vi "get_total_number_of_pixels_per_line.vi"(8 "error in (no error)":errorcluster, 11 "DL090201FrameScanTrajectory in":refnum<class "TrajectoryDL090201FrameScan.lvclass">) -> (0 "error out":errorcluster, 2 "total number of pixels per line":i32, 3 "DL090201FrameScanTrajectory out":refnum<class "TrajectoryDL090201FrameScan.lvclass">)   [LabVIEW 2010, in "TrajectoryDL090201FrameScan.lvclass"]
uses:
  TrajectoryDL090201FrameScan.lvclass
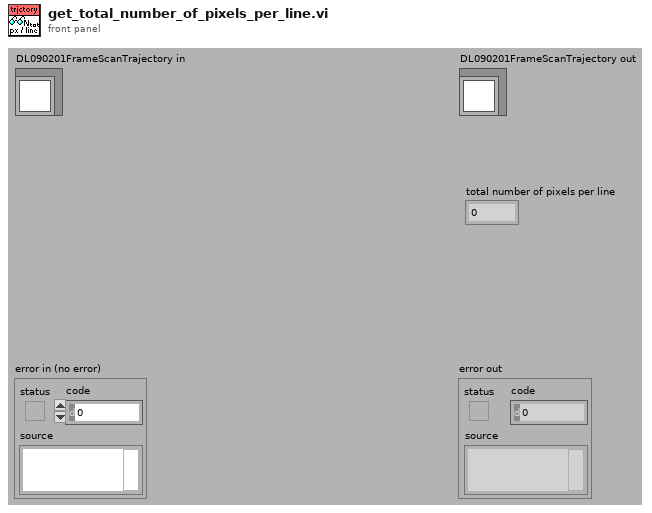
[diagram p1: front panel]
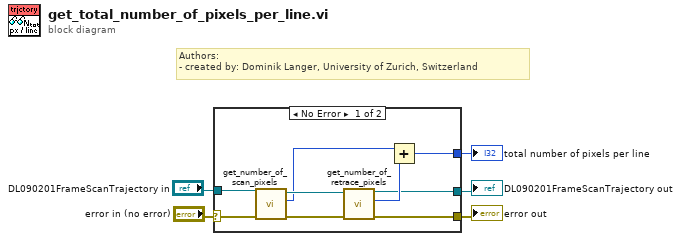
[diagram p0: block diagram]
diagram:
  # "Authors: \n- created by: Dominik Langer, University of Zurich, Switzerland"
  n1 = case shown="No Error" "error in (no error)" {
    selector: "error in (no error)" -> [w13 w16]
    tunnel: [w12 w16] -> w4
    tunnel: [w6 w15] -> w2
    tunnel: "DL090201FrameScanTrajectory in" -> [w7 w15]
    tunnel: [w8 _] -> w1
    frame No Error {
      n2 = call "get_number_of_scan_pixels.vi"("error in (no error)"=w13, "DL090201FrameScanTrajectory in"=w7) -> ("error out"=w14:errorcluster, "number of scan pixels"=w10:i32, "DL090201FrameScanTrajectory out"=w11:refnum<class "TrajectoryDL090201FrameScan.lvclass">)  [unwired: 7 out]
      n3 = call "get_number_of_retrace_pixels.vi"("error in (no error)"=w14, "DL090201FrameScanTrajectory in"=w11) -> ("error out"=w12:errorcluster, "number of retrace pixels"=w9:i32, "DL090201FrameScanTrajectory out"=w6:refnum<class "TrajectoryDL090201FrameScan.lvclass">)  [unwired: 7 out]
      n4 = Add(x=w10, y=w9) -> (x+y=w8:i32)
    }
    frame Error {
    }
  }
  "error out" <- w4
  "DL090201FrameScanTrajectory out" <- w2
  "total number of pixels per line" <- w1
